vi "click_fmv_coord.vi"(8 "error in (no error)":errorcluster, 11 "VI in":refnum<vi>) -> (0 "error out":errorcluster, 2 "Vertical":i16, 3 "Horizontal":i16)   [LabVIEW 2020, in "ui-testing.lvlib"]
uses:
  ui-testing.lvlib
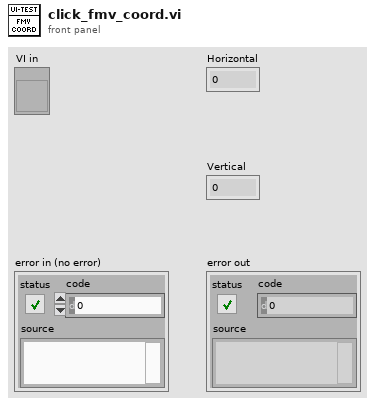
[diagram p1: front panel]
types:
  T1 = typedef "LVRectTypeDef.ctl" = cluster{"Left":i16, "Top":i16, "Right":i16, "Bottom":i16}
  T2 = typedef "LVPointTypeDef.ctl" = cluster{"Horizontal":i16, "Vertical":i16}
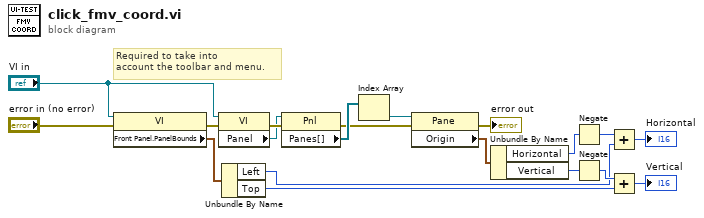
[diagram p0: block diagram]
diagram:
  # "Required to take into\naccount the toolbar and menu."
  n1 = property class="VI"(reference="VI in", error in="error in (no error)") -> (error out=w11:errorcluster, "Front Panel.PanelBounds"=w1:T1)  [unwired: 1 out]
  n2 = property class="VI"(reference="VI in", error in=w11) -> (error out=w9:errorcluster, "Panel"=w8:refnum<vi>)  [unwired: 1 out]
  n3 = Unbundle By Name(w1) -> ("Left"=w14:i16, "Top"=w16:i16)
  n4 = property class="Pnl"(reference=w8, error in=w9) -> (error out=w4:errorcluster, "Panes[]"=w5:refnum<vi>[])  [unwired: 1 out]
  n5 = Index Array(array=w5) -> (element=w6:refnum<vi>)  [unwired: 1 in]
  n6 = property class="Pane"(reference=w6, error in=w4) -> (error out=→"error out":errorcluster, "Origin"=w7:T2)  [unwired: 1 out]
  n7 = Unbundle By Name(w7) -> ("Horizontal"=w10:i16, "Vertical"=w17:i16)
  n8 = Negate(x=w10) -> (-x=w13:i16)
  n9 = Negate(x=w17) -> (-x=w19:i16)
  n10 = Add(x=w13, y=w14) -> (x+y=→"Horizontal":i16)
  n11 = Add(x=w19, y=w16) -> (x+y=→"Vertical":i16)
